vi "SET_POT.vi"(0 "TCP Network Connection in":refnum<k5>, 2 "POT_N":u32=100, 3 "VALUE":u32=100, 5 "error in (no error)":errorcluster) -> (14 "TCP Network Connection out":refnum<k5>, 15 "POT_STATUS":u8[](array[numeric]), 19 "error out":errorcluster)   [LabVIEW 2019]
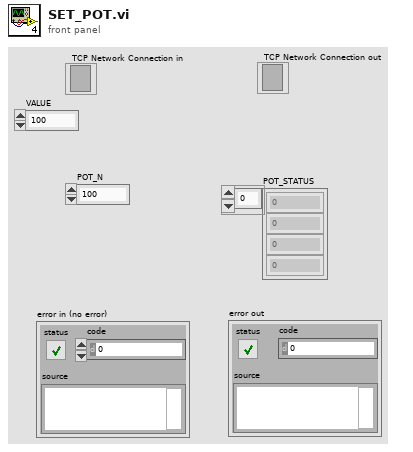
[diagram p1: front panel]
types:
  T1 = enum16{"big-endian, network order", "native, host order", "little-endian"}
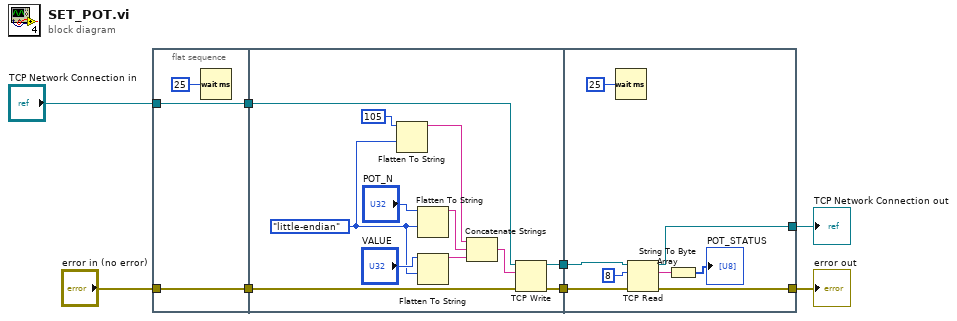
[diagram p0: block diagram]
diagram:
  n1 = flat-sequence {
    tunnel: [w10] -> w4
    tunnel: [w11] -> w3
    tunnel: "error in (no error)" -> [w11]
    tunnel: "TCP Network Connection in" -> [w10]
    tunnel: w4 -> [w23]
    tunnel: w3 -> [w22]
    tunnel: [w21] -> w2
    tunnel: [w20] -> w1
    tunnel: [w28] -> w6
    tunnel: [w29] -> w5
    tunnel: w2 -> [w31]
    tunnel: w1 -> [w30]
    frame #0 {
      n2 = Wait (ms)(milliseconds to wait=u32 25) -> ()  [unwired: 1 out]
    }
    frame #1 {
      w12 = T1."little-endian" ("byte order (0:big-endian, network order)")
      n3 = Flatten To String(anything=u32 105 ("element"), byte order (0:big-endian, network order)=w12) -> (data string=w17:string)  [unwired: 2 in, 2 out]
      n4 = Flatten To String(anything="POT_N", byte order (0:big-endian, network order)=w12) -> (data string=w19:string)  [unwired: 2 in, 2 out]
      n5 = Flatten To String(anything="VALUE", byte order (0:big-endian, network order)=w12) -> (data string=w14:string)  [unwired: 2 in, 2 out]
      n6 = Concatenate Strings(w17, w19, w14) -> (w16:string)
      n7 = TCP Write(connection ID=w23, data in=w16, error in (no error)=w22) -> (connection ID out=w21:refnum<k5>, error out=w20:errorcluster)  [unwired: 1 in, 1 out]
    }
    frame #2 {
      n8 = Wait (ms)(milliseconds to wait=u32 25) -> ()  [unwired: 1 out]
      n9 = TCP Read(connection ID=w31, bytes to read=8, error in (no error)=w30) -> (connection ID out=w29:refnum<k5>, data out=w25:string, error out=w28:errorcluster)  [unwired: 2 in]
      n10 = String To Byte Array(string=w25) -> (unsigned byte array=→"POT_STATUS":u8[])
    }
  }
  "error out" <- w6
  "TCP Network Connection out" <- w5
